vi "example.vi"() -> ()   [LabVIEW 2016]
panel:
  out "hex display":string
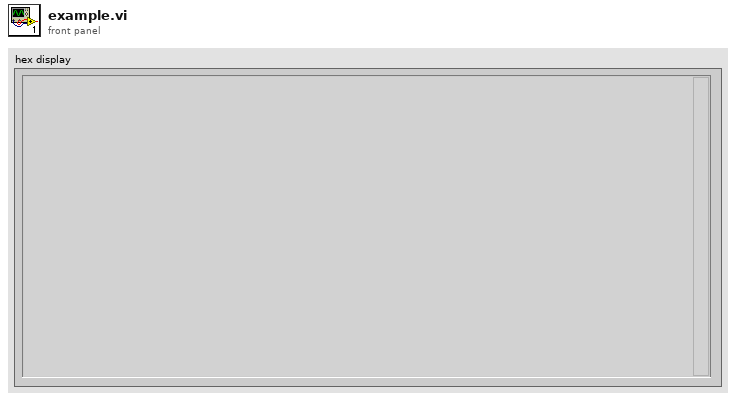
[diagram p1: front panel]
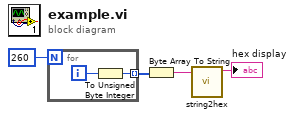
[diagram p0: block diagram]
diagram:
  n1 = for {
    N: 260 -> [_]
    tunnel: [w5] -> w3 mode=indexing
    i -> [w6]
    n2 = To Unsigned Byte Integer(number=w6) -> (unsigned 8bit integer=w5:u8)
  }
  n3 = Byte Array To String(unsigned byte array=w3) -> (string=w2:string)
  n4 = call "string2hex.vi"("data input"=w2) -> ("hex display"=→"hex display":string)  [unwired: 9 in, 1 out]
